vi "Set DAQState.vi"(8 "error in (no error)":errorcluster, 10 "DAQState Data":T1, 11 "DAQ_Engine in":refnum<class "DAQ_Engine.lvclass">) -> (0 "error out":errorcluster, 3 "DAQ_Engine out":refnum<class "DAQ_Engine.lvclass">)   [LabVIEW 2019, in "DAQ_Engine.lvclass"]
doc: "Developed by Kevin Thompson\nkevin@thompsonengineering.net\n\nCopyright 2018\nThompson Engineering, LLC"
uses:
  DAQ_Engine.lvclass
  Common/DataTypes/DAQState--enum.ctl
  DataTypes/DAQStateEvData--cluster.ctl
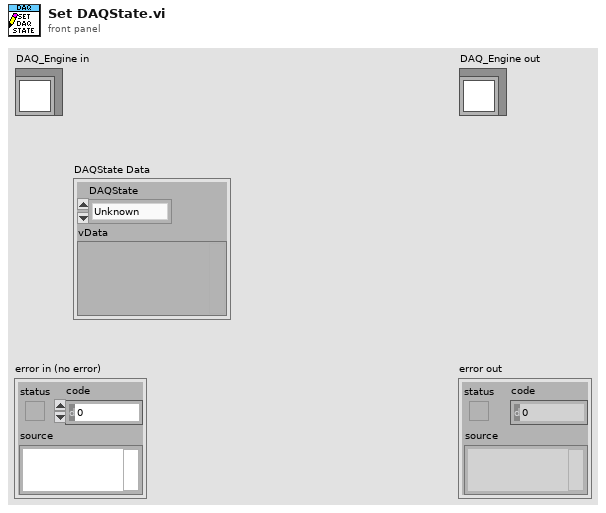
[diagram p1: front panel]
types:
  T1 = typedef "DAQ_Engine.lvclass/DAQStateEvData--cluster.ctl" = cluster{"DAQState":T2, "vData":variant}
  T2 = typedef "DAQState--enum.ctl" = enum16{"Unknown", "Stopped", "Running", "Error"}
  T3 = typedef "DAQ_Engine.lvclass/ObjData--cluster.ctl" = cluster{"Settings":T4, "Public Events":T9, "Dependency":T10, "ReadData-placeholder":T11, "VISA-placeholder":refnum<visa-resource-name>, "MeasSettings":T5, "InverterDataAcqMode":T8, "RawDaqDataQ":T12, "Private Events":T13, "DAQState Data":T1}
  T4 = typedef "DAQ_Engine.lvclass/Settings--cluster.ctl" = cluster{"Simulation":bool, "Initial ErrReporting setting":i32, "Initial Measurement settings":T5, "BoardNum":T7, "Acquisition mode":T8, "DemoMode":bool}
  T5 = typedef "Measurement Config--cluster.ctl" = cluster{"Data Rate 9775":T6, "Data Rate 9215":u32, "Samples RMS 9215":u32, "Samples RMS 9775":u32}
  T6 = typedef "nicrio_cRIO-9775_ContinuousDataRates4ChansRing.ctl" = u16
  T7 = typedef "DAQ_Engine.lvclass/BoardNum--cluster.ctl" = cluster{"P1Sgl":u32, "P2":u32, "P3":u32}
  T8 = typedef "Acquisition Mode--cluster.ctl" = enum16{"3phase", "Single"}
  T9 = typedef "DAQ_Engine.lvclass/Public Events--cluster.ctl" = cluster{"DAQ_Engine.AsyncCmd Event":refnum<user-event>, "DAQ_Engine.AsyncMsg Event":refnum<user-event>, "stop process":refnum<user-event>, "DAQ_Engine.DAQStateChg Ev":refnum<user-event>, "DAQ_Engine.MeasSettingsChg Ev":refnum<user-event>, "DAQ_Engine.AcqModeChg Ev":refnum<user-event>}
  T10 = typedef "DAQ_Engine.lvclass/Dependency--cluster.ctl" = cluster{"Config":refnum<class "Config.lvclass">}
  T11 = typedef "DAQ_Engine.lvclass/Read Data--cluster.ctl" = cluster{"Data":dbl}
  T12 = typedef "RawDAQDataQRef--cluster.ctl" = refnum<queue>
  T13 = typedef "DAQ_Engine.lvclass/Private Events--cluster.ctl" = cluster{"PrivateAsync Ev":refnum<user-event>}
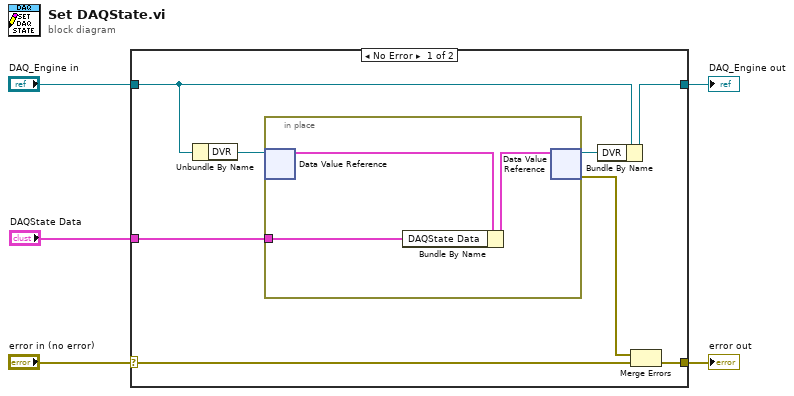
[diagram p0: block diagram]
diagram:
  n1 = case shown="No Error" "error in (no error)" {
    selector: "error in (no error)" -> [w13 w17]
    tunnel: [w7 w17] -> w4
    tunnel: [w9 w18] -> w2
    tunnel: "DAQ_Engine in" -> [w12 w18]
    tunnel: "DAQState Data" -> [w8 _]
    frame No Error {
      n2 = Unbundle By Name(w12) -> ("DVR"=w11:refnum<data-value>)
      n3 = in-place {
        in-place-border: w8 -> [w14]
        n4 = in-place-dvr #1(w11) -> (w16:T3)  [unwired: 1 out]
        n5 = Bundle By Name(cluster=w16, "DAQState Data"=w14) -> (w15:T3)
        n6 = in-place-dvr #1(w15) -> (w10:refnum<data-value>, w6:errorcluster)
      }
      n7 = Bundle By Name(cluster=w12, "DVR"=w10) -> (w9:refnum<class "DAQ_Engine.lvclass">)
      n8 = Merge Errors(w6, w13) -> (w7:errorcluster)
    }
    frame Error {
    }
  }
  "error out" <- w4
  "DAQ_Engine out" <- w2
